vi "Write Asynchronous_.vi"(8 "error in":errorcluster, 10 "Asynchronous?":bool, 11 "Module Editor Node in":refnum<class "module editor node.lvclass">) -> (0 "error out":errorcluster, 3 "Module Editor Node out":refnum<class "module editor node.lvclass">)   [LabVIEW 2013, in "PL Framework Configuration Tool.lvlib" / "module editor node.lvclass"]
uses:
  module editor node.lvclass
  module editor node.lvclass/module editor node.ctl
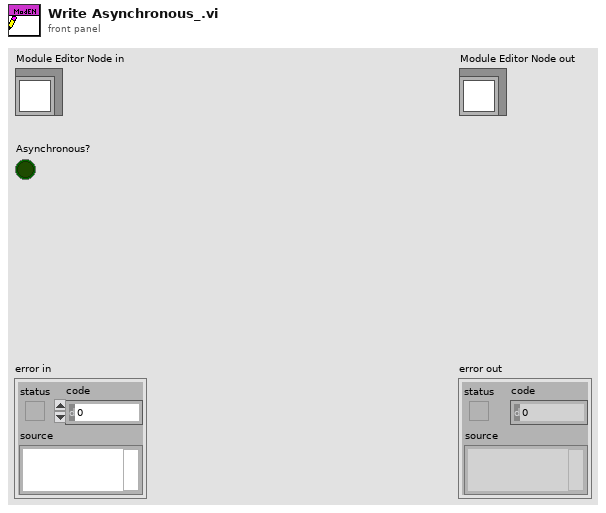
[diagram p1: front panel]
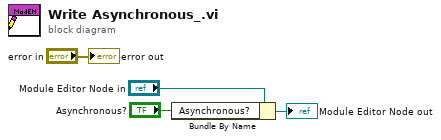
[diagram p0: block diagram]
diagram:
  n1 = Bundle By Name(cluster="Module Editor Node in", "Asynchronous?"="Asynchronous?") -> (→"Module Editor Node out":refnum<class "module editor node.lvclass">)
  "error out" <- "error in"
